vi "Create.vi"(5 "HttpDownloadTask in":refnum<class "HttpDownloadTask.lvclass">, 6 "Prefered Scale [MB]":T2=1000000 items=["Bytes"=1, "KB"=1000, "MB"=1000000, "GB"=1000000000], 8 "error in (no error)":errorcluster, 10 "FilePath":path, 11 "HttpResponseMessage":refnum<class "HttpResponseMessage.lvclass">) -> (0 "error out":errorcluster, 3 "DownloadTask Ref":T1)   [LabVIEW 2018, in "LabVIEWHTTPClient_NET.lvlib" / "HttpDownloadTask.lvclass"]
uses:
  HttpDownloadTask.lvclass
  HttpResponseMessage/HttpResponseMessage.lvclass
  Types/ScaledValue_ring.ctl
  Types/DownloadTask_ref.ctl
  Types/DownloadStats_Cluster.ctl
  HttpDownloadTask.lvclass/HttpDownloadTask.ctl
  HttpHeaders_content/HttpHeaders_Content.lvclass
  C:/Viviota/Projects/R&D/LabVIEW_HTTP_REST_NET/HTTPHeaders_NET/HttpHeaders_NET.lvclass
  LabVIEWHTTPClient_NET.lvlib
  HttpContent/HttpContent.lvclass
  HTTPHeaders_NET/HttpHeaders_NET.lvclass
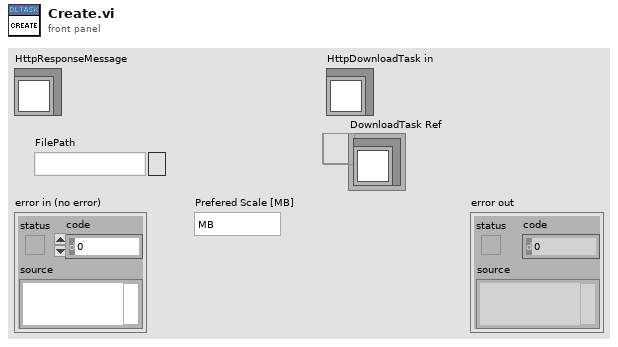
[diagram p1: front panel]
types:
  T1 = typedef "LabVIEWHTTPClient_NET.lvlib/HttpDownloadTask.lvclass/DownloadTask_ref.ctl" = refnum<data-value>
  T2 = typedef "LabVIEWHTTPClient_NET.lvlib/ScaledValue_ring.ctl" = u64
  T3 = typedef "LabVIEWHTTPClient_NET.lvlib/DownloadStats_Cluster.ctl" = cluster{"PositionCurrent":dbl, "PositionPrev":dbl, "TimeCurrent":timestamp, "TimePrev":timestamp, "TimeTotal":dbl, "PositionTotal":dbl, "TimeArray":dbl[], "PositionDifArray":dbl[], "CurrentRate":dbl, "RunningRate_10":dbl, "RunningRate":dbl, "Length":dbl}
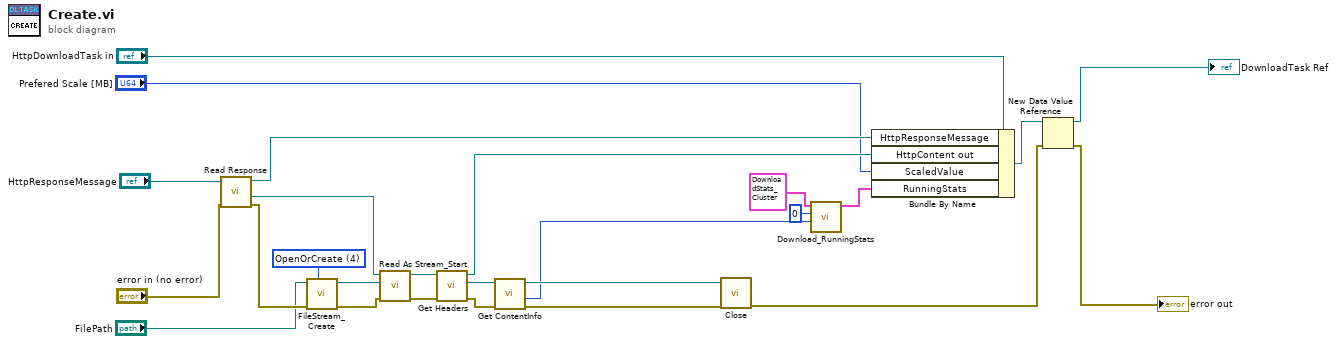
[diagram p0: block diagram]
diagram:
  w9 = 4 items=["CreateNew"=1, "Create"=2, "Open"=3, "OpenOrCreate"=4, "Truncate"=5, "Append"=6] ("mode [CreateNew]")
  n1 = call "Read Response.vi"("error in (no error)"="error in (no error)", "HttpResponseMessage in"="HttpResponseMessage") -> ("error out"=w4:errorcluster, "HttpContent out"=w5:refnum<class "HttpContent.lvclass">, "HttpResponseMessage out"=w24:refnum<class "HttpResponseMessage.lvclass">)  [unwired: 3 in, 4 out]
  n2 = call "FileStream_Create.vi"("mode [OpenOrCreate]"=w9, "error in (no error)"=w4, "FilePath"="FilePath") -> ("error out"=w10:errorcluster, "FileStream"=w8:refnum<k24>)  [unwired: 7 in]
  n3 = call "Read As Stream_Start.vi"("error in (no error)"=w10, "DestinationStream"=w8, "HttpContent in"=w5) -> ("error out"=w7:errorcluster, "HttpContent out"=w6:refnum<class "HttpContent.lvclass">)  [unwired: 7 in]
  n4 = call "Get Headers.vi"("error in (no error)"=w7, "HttpContent in"=w6) -> ("error out"=w21:errorcluster, "HTTPHeaders"=w22:refnum<class "HttpHeaders_Content.lvclass">, "HttpContent out"=w18:refnum<class "HttpContent.lvclass">)  [unwired: 7 in]
  n5 = call "Get ContentInfo.vi"("error in (no error)"=w21, "HttpHeaders_Content in"=w22) -> ("error out"=w20:errorcluster, "Length"=w15:i64, "HttpHeaders_Content out"=w19:refnum<class "HttpHeaders_Content.lvclass">)  [unwired: 6 in, 1 out]
  n6 = call "Close.vi"("error in (no error)"=w20, "HTTPHeaders_NET in"=w19) -> ("error out"=w13:errorcluster)  [unwired: 9 in]
  n7 = call "Download_RunningStats.vi"("Length"=w15, "Position"=i64 0, "DownloadStats In"=T3 {"PositionCurrent"=0.0, "PositionPrev"=0.0, "TimeCurrent"=timestamp(0 s since 1904-01-01), "TimePrev"=timestamp(0 s since 1904-01-01), "TimeTotal"=0.0, "PositionTotal"=0.0, "TimeArray"=[], "PositionDifArray"=[], "CurrentRate"=0.0, "RunningRate_10"=0.0, "RunningRate"=0.0, "Length"=0.0} ("RunningStats")) -> ("RunningStats"=w16:T3)  [unwired: 8 in]
  n8 = Bundle By Name(cluster="HttpDownloadTask in", "HttpResponseMessage"=w24, "HttpContent out"=w18, "ScaledValue"="Prefered Scale [MB]", "RunningStats"=w16) -> (w2:refnum<class "HttpDownloadTask.lvclass">)
  n9 = New Data Value Reference(data value=w2, error in=w13) -> (data value reference=→"DownloadTask Ref":refnum<data-value>, error out=→"error out":errorcluster)
